vi "ReceiveCommand.vi"(8 "error in (no error)":errorcluster, 11 "OXY_SCPI Reseource In":refnum<visa-resource-name>) -> (0 "error out":errorcluster, 1 "received Data with Header":string, 2 "received Data":string, 3 "OXY_SCPI Reseource Out":refnum<visa-resource-name>)   [LabVIEW 2020, in "OXYGEN_Datastream.lvlib"]
uses:
  OXYGEN_Datastream.lvlib
  TypeDefs/Modes_FGV_OutputHeaderFormat.ctl
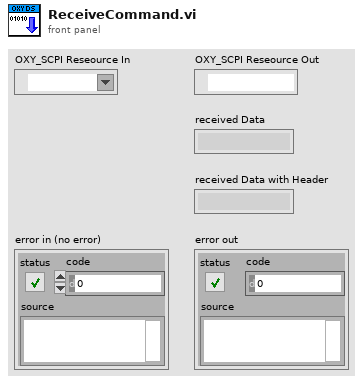
[diagram p1: front panel]
types:
  T1 = typedef "OXYGEN_Datastream.lvlib/Modes_FGV_OutputHeaderFormat.ctl" = enum16{"Set", "Get"}
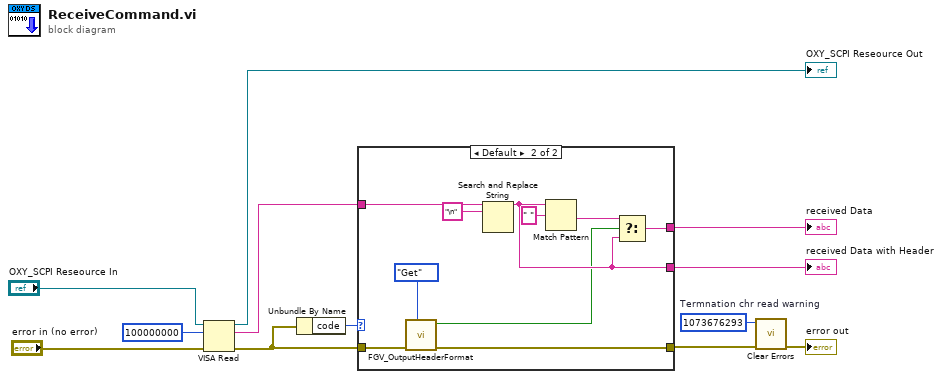
[diagram p0: block diagram]
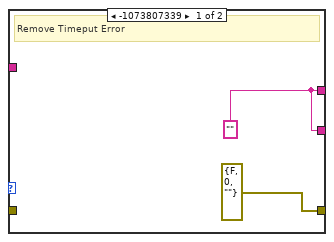
[diagram p2: hidden frame]
diagram:
  w3 = 1073676293  # Termnation chr read warning
  n1 = VISA Read(VISA resource name="OXY_SCPI Reseource In", byte count=u32 100000000, error in (no error)="error in (no error)") -> (VISA resource name out=→"OXY_SCPI Reseource Out":refnum<visa-resource-name>, read buffer=w8:string, error out=w5:errorcluster)  [unwired: 1 out]
  n2 = Unbundle By Name(w5) -> ("code"=w6:i32)
  n3 = case shown="Default" w6 {
    tunnel: w8 -> [_ w24]
    tunnel: [w13 w20] -> w7
    tunnel: [errorcluster {"status"=FALSE, "code"=0, "source"=""} ("error out") w17] -> w2
    tunnel: w5 -> [_ w18]
    tunnel: [w13 w19] -> w4
    frame -1073807339 {
      w13 = "" ("result string")
      # "Remove Timeput Error"
    }
    frame Default {
      n4 = call "FGV_OutputHeaderFormat.vi"("Mode"=Modes_FGV_OutputHeaderFormat."Get", "error in (no error)"=w18) -> ("error out"=w17:errorcluster, "Header On?"=w16:bool)  [unwired: 7 in, 1 out]
      n5 = Search and Replace String(input string=w24, search string="\n") -> (result string=w19:string)  [unwired: 6 in, 3 out]
      n6 = Match Pattern(string=w19, regular expression=" ") -> (after substring=w21:string)  [unwired: 1 in, 3 out]
      n7 = Select(t=w21, s=w16, f=w19) -> (s? t:f=w20:string)
    }
  }
  "received Data" <- w7
  "received Data with Header" <- w4
  n8 = call <vilib>:"Clear Errors.vi"("error in (no error)"=w2, "specific error code to clear (0: all)"=w3) -> ("error out"=→"error out":errorcluster)  [unwired: 4 in, 1 out]
